vi "Parse_array_settings.vi"(8 "error in (no error)":errorcluster, 11 "Value":string) -> (0 "error out":errorcluster, 3 "Array":dbl[](array[numeric]))   [LabVIEW 2020, in "Config.lvclass"]
uses:
  Config/Config.lvclass
  <vilib>/regexp/Match Regular Expression.xnode
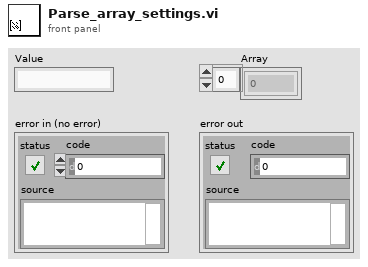
[diagram p1: front panel]
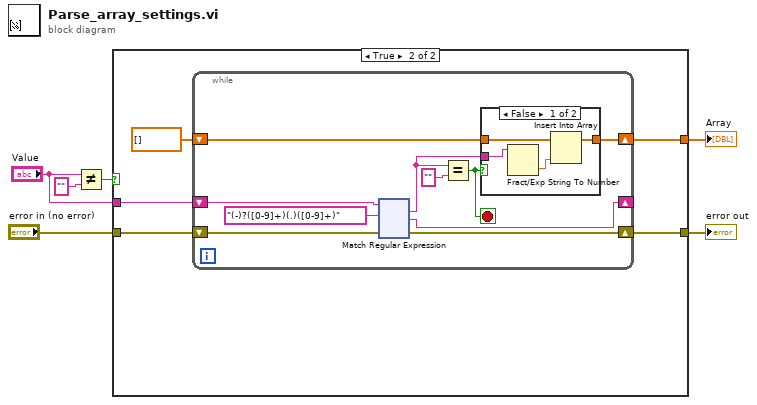
[diagram p0: block diagram]
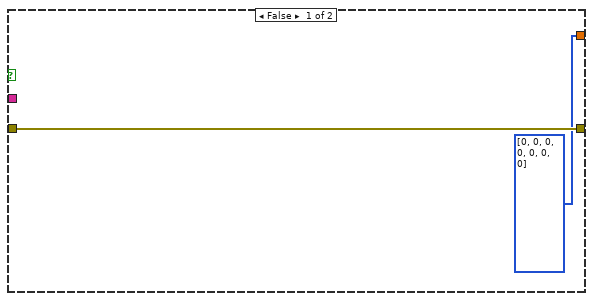
[diagram p2: hidden frame]
diagram:
  n1 = Not Equal?(x="Value", y="") -> (x != y?=w2:bool)
  n2 = case shown="True" w2 {
    tunnel: "error in (no error)" -> [w8 w13]
    tunnel: [w8 w12] -> w4
    tunnel: "Value" -> [_ w11]
    tunnel: [i32[] [0, 0, 0, 0, 0, 0, 0] ("Array") w9] -> w6
    frame False {
    }
    frame True {
      n3 = while {
        shift-right: [w22] -> _
        shift-left: w11 -> [w23]
        shift-right: [w17] -> w9
        shift-left: dbl[] [] ("Array") -> [w16]
        shift-right: [w14] -> w12
        shift-left: w13 -> [w15]
        stop <- w18 stop-if-true
        n4 = xnode "Match Regular Expression"("input string"=w23, "regular expression"="(-)?([0-9]+)(.)([0-9]+)", "error in"=w15) -> ("whole match"=w20:string, "after match"=w22:string, "error out"=w14:errorcluster)  [unwired: 3 in, 2 out]
        n5 = Equal?(x=w20, y="") -> (x = y?=w18:bool)
        n6 = case shown="False" w18 {
          tunnel: w20 -> [w25 _]
          tunnel: [w26 w28] -> w17
          tunnel: w16 -> [w27 w28]
          frame False {
            n7 = Fract/Exp String To Number(string=w25) -> (number=w24:dbl)  [unwired: 3 in, 1 out]
            n8 = Insert Into Array(array=w27, new element=w24) -> (w26:dbl[])  [unwired: 1 in]
          }
          frame True {
          }
        }
      }
    }
  }
  "Array" <- w6
  "error out" <- w4
